vi "ob.cmd.to.str.vi"(11 "orderbook.command":T1={"type"=enum."AddOrder", "side"=66, "orderId "=12593, "quantity"=100, "symbol"=0, "price"=10025, "executed.qty"=125, "canceled.qty"=0, "remaining.qty"=0, "seconds"=0, "nanoseconds"=1234, "Add"=TRUE, "Edit"=FALSE, "Remove"=FALSE, "seq no"=15, "recv.time"=100, "parse.time"=150} {"orderId" format="%.0x"; "side" format="%.0x"}) -> (3 "string":string)   [LabVIEW 2020, in "fpganow.common.host.lvlib"]
uses:
  fpganow.common.host.lvlib
  fpga/orderbook.command.ctl
  fpga/orderbook.command.type.ctl
  fpga/fpganow.common.fpga.lvlib
panel:
  out "unsigned byte array":u8[](array[numeric])=[79, 82, 68, 48, 48, 49] format="%.0x"
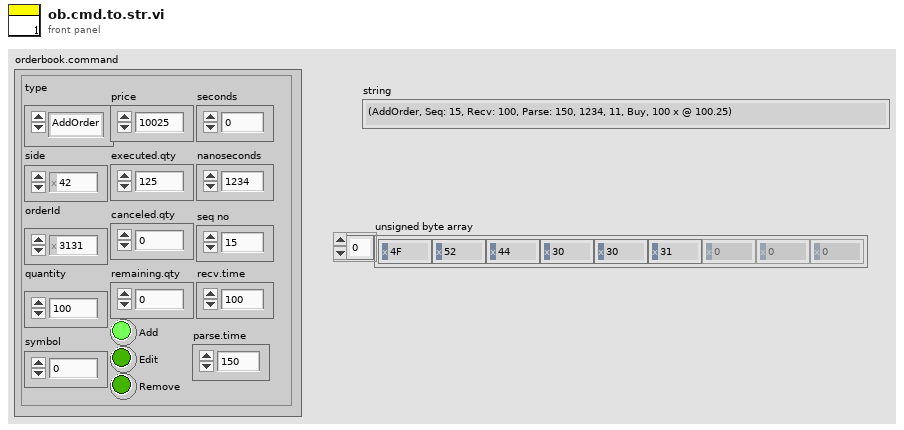
[diagram p1: front panel]
types:
  T1 = typedef "fpganow.common.fpga.lvlib/orderbook.command.ctl" = cluster{"type":T2, "side":u8, "orderId ":u64, "quantity":u32, "symbol":u64, "price":u64, "executed.qty":u32, "canceled.qty":u32, "remaining.qty":u32, "seconds":u64, "nanoseconds":u64, "Add":bool, "Edit":bool, "Remove":bool, "seq no":u32, "recv.time":u64, "parse.time":u64}
  T2 = typedef "fpganow.common.fpga.lvlib/orderbook.command.type.ctl" = enum8{"Time", "AddOrder", "OrderExecuted", "OrderExecutedAtPrice", "ReduceSize", "ModifyOrder", "DeleteOrder", "Get.Everything", "Get.All.Orders", "Get.Top"}
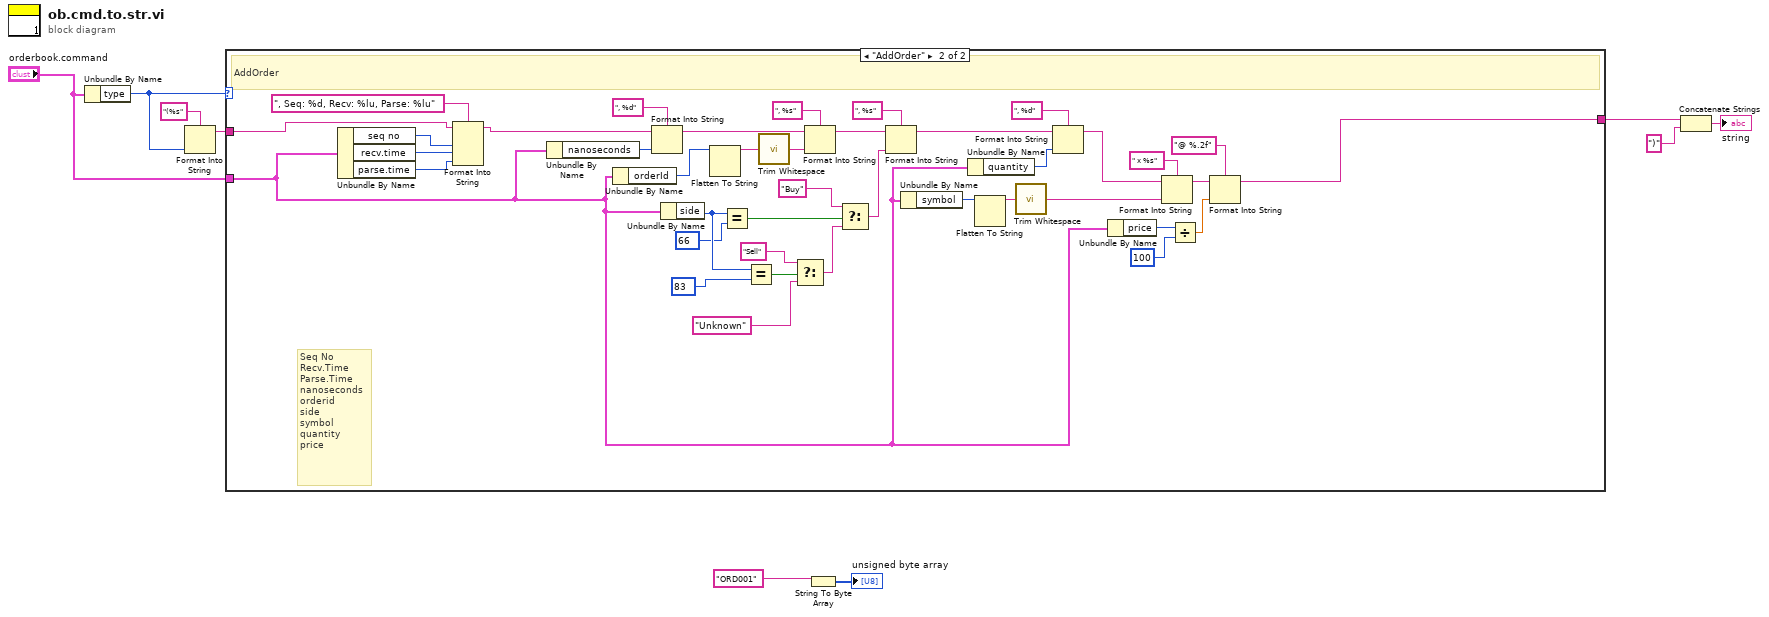
[diagram p0: block diagram]
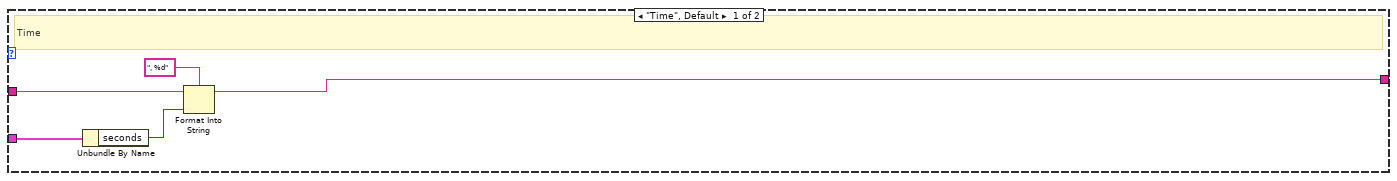
[diagram p2: hidden frame]
diagram:
  n1 = Unbundle By Name("orderbook.command") -> ("type"=w3:T2)
  n2 = Format Into String(format string="(%s", w3) -> (resulting string=w5:string)  [unwired: 2 in, 1 out]
  n3 = case shown="\"AddOrder\"" w3 {
    tunnel: "orderbook.command" -> [w14 w19]
    tunnel: [w10 w31] -> w7
    tunnel: w5 -> [w11 w15]
    frame "Time", Default {
      # "Time"
      n4 = Unbundle By Name(w14) -> ("seconds"=w13:u64)
      n5 = Format Into String(format string=", %d", initial string=w11, w13) -> (resulting string=w10:string)  [unwired: 1 in, 1 out]
    }
    frame "AddOrder" {
      # "Seq No\nRecv.Time\nParse.Time\nnanoseconds\norderid\nside\nsymbol\nquantity\nprice"
      # "AddOrder"
      n6 = Unbundle By Name(w19) -> ("seq no"=w21:u32, "recv.time"=w18:u64, "parse.time"=w17:u64)
      n7 = Format Into String(format string=", Seq: %d, Recv: %lu, Parse: %lu", initial string=w15, w21, w18, w17) -> (resulting string=w16:string)  [unwired: 1 in, 1 out]
      n8 = Unbundle By Name(w19) -> ("nanoseconds"=w54:u64)
      n9 = Unbundle By Name(w19) -> ("orderId"=w22:u64)
      n10 = Format Into String(format string=", %d", initial string=w16, w54) -> (resulting string=w51:string)  [unwired: 1 in, 1 out]
      n11 = Unbundle By Name(w19) -> ("side"=w48:u8)
      n12 = Flatten To String(anything=w22) -> (data string=w24:string)  [unwired: 3 in, 2 out]
      n13 = Equal?(x=w48, y=u8 66) -> (x = y?=w42:bool)
      n14 = Equal?(x=w48, y=u8 83) -> (x = y?=w49:bool)
      n15 = call <vilib>:"Trim Whitespace.vi"("string"=w24) -> ("trimmed string"=w23:string)  [unwired: 1 in]
      n16 = Select(t="Sell", s=w49, f="Unknown") -> (s? t:f=w50:string)
      n17 = Format Into String(format string=", %s", initial string=w51, w23) -> (resulting string=w41:string)  [unwired: 1 in, 1 out]
      n18 = Select(t="Buy", s=w42, f=w50) -> (s? t:f=w40:string)
      n19 = Format Into String(format string=", %s", initial string=w41, w40) -> (resulting string=w29:string)  [unwired: 1 in, 1 out]
      n20 = Unbundle By Name(w19) -> ("symbol"=w27:u64)
      n21 = Unbundle By Name(w19) -> ("quantity"=w37:u32)
      n22 = Flatten To String(anything=w27) -> (data string=w26:string)  [unwired: 3 in, 2 out]
      n23 = call <vilib>:"Trim Whitespace.vi"("string"=w26) -> ("trimmed string"=w25:string)  [unwired: 1 in]
      n24 = Format Into String(format string=", %d", initial string=w29, w37) -> (resulting string=w28:string)  [unwired: 1 in, 1 out]
      n25 = Unbundle By Name(w19) -> ("price"=w34:u64)
      n26 = Format Into String(format string=" x %s", initial string=w28, w25) -> (resulting string=w30:string)  [unwired: 1 in, 1 out]
      n27 = Divide(x=w34, y=u64 100) -> (x/y=w32:dbl)
      n28 = Format Into String(format string="@ %.2f", initial string=w30, w32) -> (resulting string=w31:string)  [unwired: 1 in, 1 out]
    }
  }
  n29 = String To Byte Array(string="ORD001") -> (unsigned byte array=→"unsigned byte array":u8[])
  n30 = Concatenate Strings(w7, ")") -> (→"string":string)
